vi "Test DAQmx.vi"() -> ()   [LabVIEW 2020, in "DAQmx.lvclass"]
uses:
  DAQmx.lvclass
  typedefs/DAQ.Config.AO--Cluster--Array.ctl
  typedefs/DAQ.Config.AO--Cluster.ctl
  typedefs/DAQ.Config.AO.Range--enum.ctl
  typedefs/DAQ.Config.Device Type--enum.ctl
  typedefs/DAQ.Config.AI--Cluster--Array.ctl
  typedefs/DAQ.Config.AI--Cluster.ctl
  typedefs/DAQ.Config.AI.Coupling--enum.ctl
  typedefs/DAQ.Config.AI.Range--enum.ctl
  typedefs/DAQ.Config.Timing.Sampling--Cluster.ctl
  DAQmx.lvclass/DAQmx.ctl
panel:
  in  "single device":bool
  in  "Sampling":T1={"Fs"=52000.0, "#s"=5000} {"Fs" format="%#_13g"}
  in  "AI":T2=[{"Channels"="PXI1Slot3/ai0", "Coupling"=10050, "Range"=enum."±0.316", "input terminal configuration"=-1, "Type"=enum."None"}, {"Channels"="PXI1Slot3/ai1", "Coupling"=10050, "Range"=enum."±0.316", "input terminal configuration"=-1, "Type"=enum."None"}, {"Channels"="PXI1Slot5/ai0", "Coupling"=10050, "Range"=enum."±0.316", "input terminal configuration"=-1, "Type"=enum."None"}, {"Channels"="PXI1Slot5/ai1", "Coupling"=10050, "Range"=enum."±0.316", "input terminal configuration"=-1, "Type"=enum."None"}] {"input terminal configuration" items=[""=-1, "Differential"=10106, "Pseudodifferential"=12529]; "Coupling" items=[""=0, "AC"=10045, "DC"=10050, "GND"=10066]}
  in  "AO":T7=[{"Channels"="PXI1Slot3/ao0", "Range"=enum."±1.0", "output terminal configuration"=-1, "Type"=enum."None"}, {"Channels"="PXI1Slot3/ao1", "Range"=enum."±1.0", "output terminal configuration"=-1, "Type"=enum."None"}, {"Channels"="PXI1Slot5/ao0", "Range"=enum."±1.0", "output terminal configuration"=-1, "Type"=enum."None"}, {"Channels"="PXI1Slot5/ao1", "Range"=enum."±1.0", "output terminal configuration"=-1, "Type"=enum."None"}] {"output terminal configuration" items=[""=-1, "Differential"=10106, "Pseudodifferential"=12529]}
  out "error out":errorcluster
  out "Waveform Graph":waveform(dbl)[](graph)
  in  "stop":bool
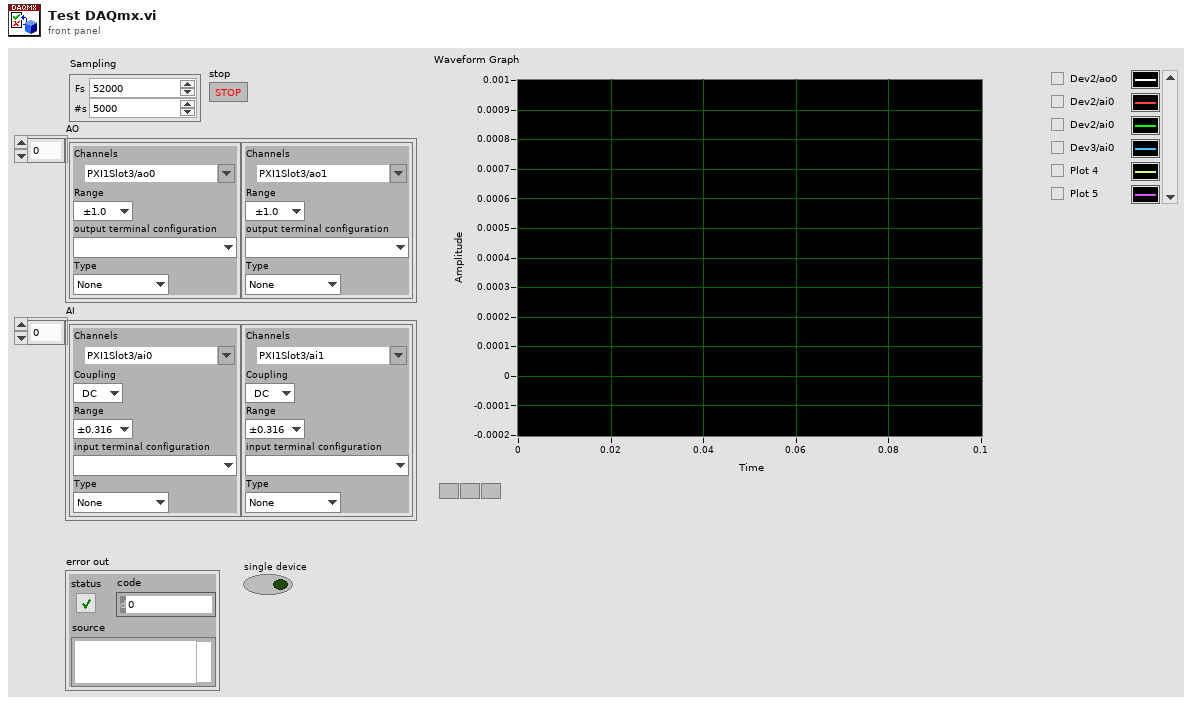
[diagram p1: front panel]
types:
  T1 = typedef "DAQmx.lvclass/DAQ.Config.Timing.Sampling--Cluster.ctl" = cluster{"Fs":dbl, "#s":i32}
  T2 = typedef "DAQmx.lvclass/DAQ.Config.AI--Cluster--Array.ctl" = T3[]
  T3 = typedef "DAQmx.lvclass/DAQ.Config.AI--Cluster.ctl" = cluster{"Channels":tag, "Coupling":T4, "Range":T5, "input terminal configuration":i32, "Type":T6}
  T4 = typedef "DAQmx.lvclass/DAQ.Config.AI.Coupling--enum.ctl" = u16
  T5 = typedef "DAQmx.lvclass/DAQ.Config.AI.Range--enum.ctl" = enum16{"±0.316", "±1.00", "±3.16", "±10.0", "±31.6", "±42.4", ""}
  T6 = typedef "DAQmx.lvclass/DAQ.Config.Device Type--enum.ctl" = enum16{"None", "USB-4431", "PXI-446x"}
  T7 = typedef "DAQmx.lvclass/DAQ.Config.AO--Cluster--Array.ctl" = T8[]
  T8 = typedef "DAQmx.lvclass/DAQ.Config.AO--Cluster.ctl" = cluster{"Channels":tag, "Range":T9, "output terminal configuration":i32, "Type":T6}
  T9 = typedef "DAQmx.lvclass/DAQ.Config.AO.Range--enum.ctl" = enum16{"±0.1", "±1.0", "±10.0", ""}
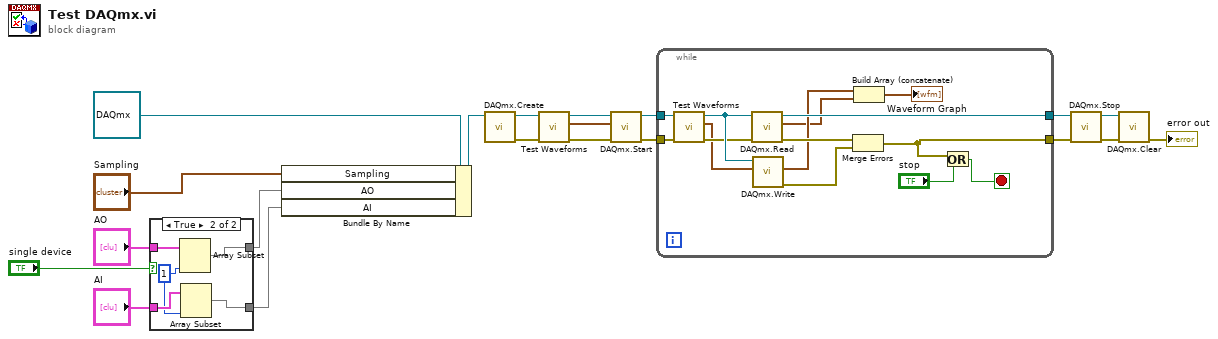
[diagram p0: block diagram]
diagram:
  n1 = case shown="True" "single device" {
    tunnel: [w22 w26] -> w4
    tunnel: "AO" -> [w22 w27]
    tunnel: [w21 w24] -> w2
    tunnel: "AI" -> [w21 w25]
    frame False {
    }
    frame True {
      w23 = 1 ("length")
      n2 = Array Subset(array=w27, length=w23) -> (w26:T7)  [unwired: 1 in]
      n3 = Array Subset(array=w25, length=w23) -> (w24:T2)  [unwired: 1 in]
    }
  }
  n4 = Bundle By Name(cluster=refnum<class "DAQmx.lvclass"> refnum ("DAQmx in"), "Sampling"="Sampling", "AO"=w4, "AI"=w2) -> (w20:refnum<class "DAQmx.lvclass">)
  n5 = call "DAQmx.Create.vi"("DAQmx in"=w20) -> ("error out"=w9:errorcluster, "DAQmx out"=w12:refnum<class "DAQmx.lvclass">)  [unwired: 9 in]
  n6 = call "Test Waveforms.vi"("error in (no error)"=w9, "DAQmx in"=w12) -> ("error out"=w10:errorcluster, "Array"=w8:waveform(dbl)[], "DAQmx out"=w11:refnum<class "DAQmx.lvclass">)  [unwired: 7 in]
  n7 = call "DAQmx.Start.vi"("error in"=w10, "WFM in"=w8, "DAQmx in"=w11) -> ("error out"=w14:errorcluster, "DAQmx out"=w19:refnum<class "DAQmx.lvclass">)  [unwired: 7 in]
  n8 = while {
    tunnel: w19 -> [w35]
    tunnel: [w41] -> w18
    tunnel: [w36] -> w15
    tunnel: w14 -> [w33]
    stop <- w37 stop-if-true
    n9 = call "Test Waveforms.vi"("error in (no error)"=w33, "DAQmx in"=w35) -> ("error out"=w32:errorcluster, "Array"=w30:waveform(dbl)[], "DAQmx out"=w34:refnum<class "DAQmx.lvclass">)  [unwired: 7 in]
    n10 = call "DAQmx.Read.vi"("error in"=w32, "DAQmx in"=w34) -> ("error out"=w40:errorcluster, "AIwfm"=w28:waveform(dbl)[], "DAQmx out"=w41:refnum<class "DAQmx.lvclass">)  [unwired: 6 in, 1 out]
    n11 = call "DAQmx.Write.vi"("AOwfm"=w30, "DAQmx in"=w34) -> ("error out"=w31:errorcluster, "AOwfm out (previous)"=w29:waveform(dbl)[])  [unwired: 6 in, 2 out]
    n12 = Merge Errors(w40, w31) -> (w36:errorcluster)
    n13 = Build Array (concatenate)(w29, w28) -> (→"Waveform Graph":waveform(dbl)[])
    n14 = Or(x=w36, y="stop") -> (x .or. y?=w37:bool)
  }
  n15 = call "DAQmx.Stop.vi"("error in (no error)"=w15, "DAQmx in"=w18) -> ("error out"=w16:errorcluster, "DAQmx out"=w17:refnum<class "DAQmx.lvclass">)  [unwired: 8 in]
  n16 = call "DAQmx.Clear.vi"("error in (no error)"=w16, "DAQmx in"=w17) -> ("error out"=→"error out":errorcluster)  [unwired: 8 in, 1 out]
